vi "Data Storage - Pack Elements (B256).vi"(0 "data in":bool[](array[boolean]), 2 "reset":bool, 5 "input valid":bool, 7 "bit count":u16, 12 "ready for output (T)":bool=TRUE) -> (4 "data out":bool[](array[boolean]), 6 "output valid":bool, 14 "ready for input":bool)   [LabVIEW 2018, in "Streaming FPGA.lvlib"]
doc: "Packs arrays of booleans into arrays of 256 booleans.\n\nEach input array can have a different number of valid elements between 0 and 256, while the output array has always 256 valid elements. This VI reads <B>bit count</B> number of elements from the <B>data in</B> input array starting from the first element of the array, and returns them in arrays of 256 elements."
uses:
  Streaming FPGA.lvlib
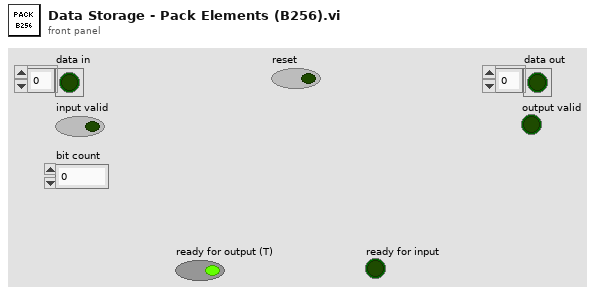
[diagram p1: front panel]
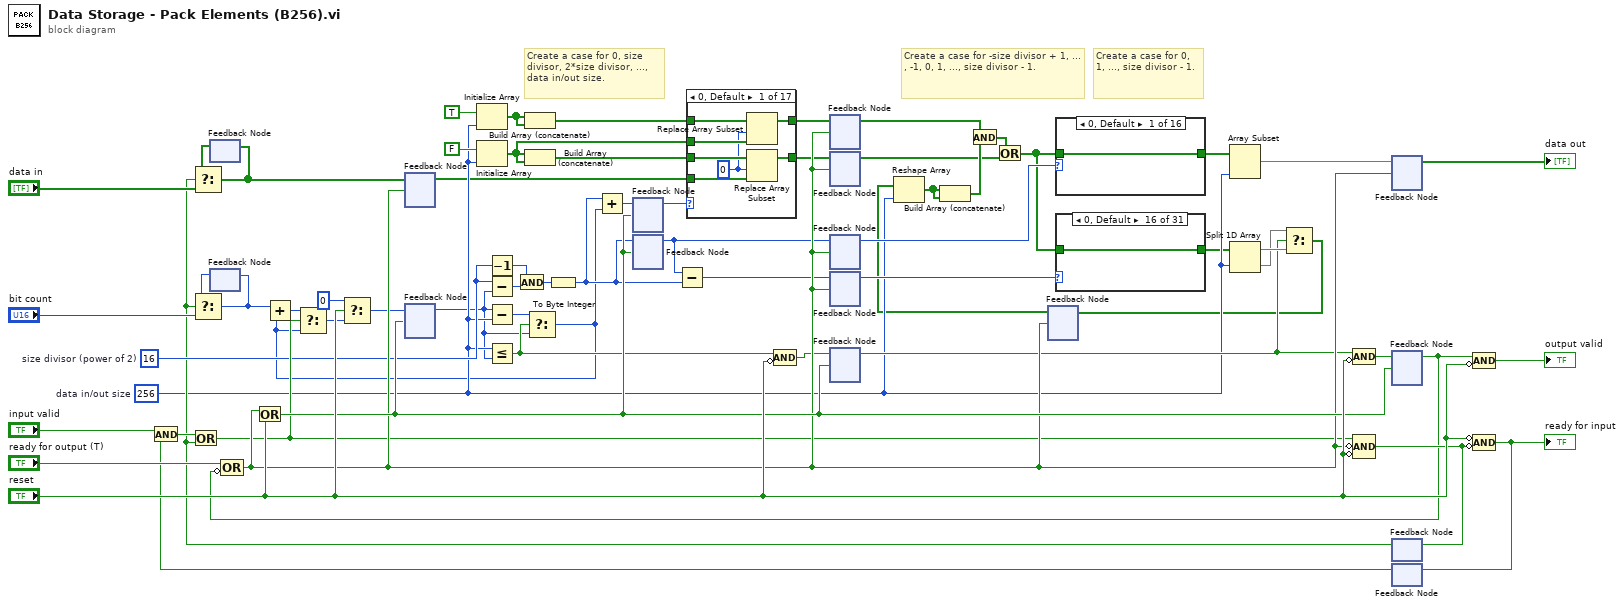
[diagram p0: block diagram]
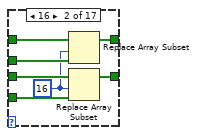
[diagram p2: hidden frame]
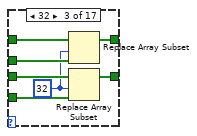
[diagram p3: hidden frame]
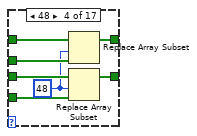
[diagram p4: hidden frame]
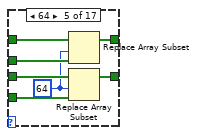
[diagram p5: hidden frame]
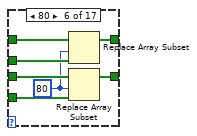
[diagram p6: hidden frame]
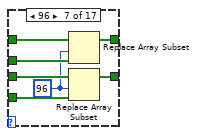
[diagram p7: hidden frame]
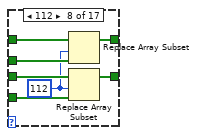
[diagram p8: hidden frame]
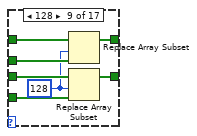
[diagram p9: hidden frame]
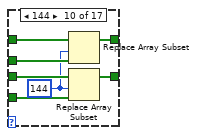
[diagram p10: hidden frame]
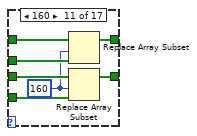
[diagram p11: hidden frame]
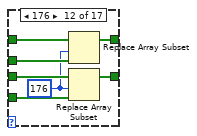
[diagram p12: hidden frame]
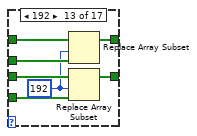
[diagram p13: hidden frame]
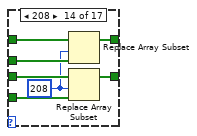
[diagram p14: hidden frame]
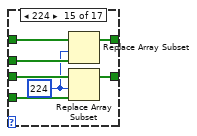
[diagram p15: hidden frame]
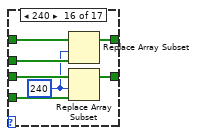
[diagram p16: hidden frame]
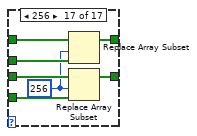
[diagram p17: hidden frame]
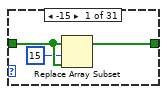
[diagram p18: hidden frame]
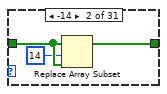
[diagram p19: hidden frame]
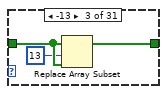
[diagram p20: hidden frame]
diagram:
  w52 = u16 16  # size divisor (power of 2)
  w27 = u16 256  # data in/out size
  # "Create a case for 0, 1, ..., size divisor - 1."
  # "Create a case for -size divisor + 1, ..., -1, 0, 1, ..., size divisor - 1."
  # "Create a case for 0, size divisor, 2*size divisor, ..., data in/out size."
  n1 = feedback #1() -> (w59:bool[])  [unwired: 1 in]
  n2 = feedback #2() -> (w56:u16)  [unwired: 1 in]
  n3 = feedback #3() -> (w4:bool[])  [unwired: 1 in]
  n4 = feedback #4() -> (w7:u16)  [unwired: 1 in]
  n5 = Initialize Array(TRUE ("element"), w27) -> (w24:bool[])
  n6 = Initialize Array(FALSE, w27) -> (w21:bool[])
  n7 = Decrement(x=w52) -> (x-1=w54:u16)
  n8 = Subtract(x=w52, y=w7) -> (x-y=w55:u16)
  n9 = Subtract(x=w7, y=w27) -> (x-y=w61:u16)
  n10 = Less Or Equal?(x=w27, y=w7) -> (x <= y?=w40:bool)
  n11 = And(x=w54, y=w55) -> (x .and. y?=w47:u16)
  n12 = Build Array (concatenate)(w24, w24) -> (w22:bool[])
  n13 = Build Array (concatenate)(w21, w21) -> (w23:bool[])
  n14 = Select(t=w61, s=w40, f=w7) -> (s? t:f=w6:u16)
  n15 = To Byte Integer(number=w47) -> (8bit integer=w12:i8)
  n16 = Add(x=w12, y=w6) -> (x+y=w11:u16)
  n17 = feedback #5() -> (w25:u16)  [unwired: 1 in]
  n18 = feedback #6() -> (w42:i8)  [unwired: 1 in]
  n19 = Subtract(x=w42, y=w12) -> (x-y=w44:i8)
  n20 = case shown="0, Default" w25 {
    tunnel: w23 -> [w72 w79 w86 w93 w100 w107 w114 w121 w128 w135 w142 w149 w156 w163 w170 w177 w184]
    tunnel: w4 -> [w71 w78 w85 w92 w99 w106 w113 w120 w127 w134 w141 w148 w155 w162 w169 w176 w183]
    tunnel: [w70 w77 w84 w91 w98 w105 w112 w119 w126 w133 w140 w147 w154 w161 w168 w175 w182] -> w20
    tunnel: w22 -> [w69 w76 w83 w90 w97 w104 w111 w118 w125 w132 w139 w146 w153 w160 w167 w174 w181]
    tunnel: w21 -> [w68 w75 w82 w89 w96 w103 w110 w117 w124 w131 w138 w145 w152 w159 w166 w173 w180]
    tunnel: [w66 w73 w80 w87 w94 w101 w108 w115 w122 w129 w136 w143 w150 w157 w164 w171 w178] -> w19
    frame 0, Default {
      w67 = 0 ("index")
      n21 = Replace Array Subset(array=w69, new element=w68, index=w67) -> (w66:bool[])
      n22 = Replace Array Subset(array=w72, new element=w71, index=w67) -> (w70:bool[])
    }
    frame 16 {
      w74 = 16 ("index")
      n23 = Replace Array Subset(array=w76, new element=w75, index=w74) -> (w73:bool[])
      n24 = Replace Array Subset(array=w79, new element=w78, index=w74) -> (w77:bool[])
    }
    frame 32 {
      w81 = 32 ("index")
      n25 = Replace Array Subset(array=w83, new element=w82, index=w81) -> (w80:bool[])
      n26 = Replace Array Subset(array=w86, new element=w85, index=w81) -> (w84:bool[])
    }
    frame 48 {
      w88 = 48 ("index")
      n27 = Replace Array Subset(array=w90, new element=w89, index=w88) -> (w87:bool[])
      n28 = Replace Array Subset(array=w93, new element=w92, index=w88) -> (w91:bool[])
    }
    frame 64 {
      w95 = 64 ("index")
      n29 = Replace Array Subset(array=w97, new element=w96, index=w95) -> (w94:bool[])
      n30 = Replace Array Subset(array=w100, new element=w99, index=w95) -> (w98:bool[])
    }
    frame 80 {
      w102 = 80 ("index")
      n31 = Replace Array Subset(array=w104, new element=w103, index=w102) -> (w101:bool[])
      n32 = Replace Array Subset(array=w107, new element=w106, index=w102) -> (w105:bool[])
    }
    frame 96 {
      w109 = 96 ("index")
      n33 = Replace Array Subset(array=w111, new element=w110, index=w109) -> (w108:bool[])
      n34 = Replace Array Subset(array=w114, new element=w113, index=w109) -> (w112:bool[])
    }
    frame 112 {
      w116 = 112 ("index")
      n35 = Replace Array Subset(array=w118, new element=w117, index=w116) -> (w115:bool[])
      n36 = Replace Array Subset(array=w121, new element=w120, index=w116) -> (w119:bool[])
    }
    frame 128 {
      w123 = 128 ("index")
      n37 = Replace Array Subset(array=w125, new element=w124, index=w123) -> (w122:bool[])
      n38 = Replace Array Subset(array=w128, new element=w127, index=w123) -> (w126:bool[])
    }
    frame 144 {
      w130 = 144 ("index")
      n39 = Replace Array Subset(array=w132, new element=w131, index=w130) -> (w129:bool[])
      n40 = Replace Array Subset(array=w135, new element=w134, index=w130) -> (w133:bool[])
    }
    frame 160 {
      w137 = 160 ("index")
      n41 = Replace Array Subset(array=w139, new element=w138, index=w137) -> (w136:bool[])
      n42 = Replace Array Subset(array=w142, new element=w141, index=w137) -> (w140:bool[])
    }
    frame 176 {
      w144 = 176 ("index")
      n43 = Replace Array Subset(array=w146, new element=w145, index=w144) -> (w143:bool[])
      n44 = Replace Array Subset(array=w149, new element=w148, index=w144) -> (w147:bool[])
    }
    frame 192 {
      w151 = 192 ("index")
      n45 = Replace Array Subset(array=w153, new element=w152, index=w151) -> (w150:bool[])
      n46 = Replace Array Subset(array=w156, new element=w155, index=w151) -> (w154:bool[])
    }
    frame 208 {
      w158 = 208 ("index")
      n47 = Replace Array Subset(array=w160, new element=w159, index=w158) -> (w157:bool[])
      n48 = Replace Array Subset(array=w163, new element=w162, index=w158) -> (w161:bool[])
    }
    frame 224 {
      w165 = 224 ("index")
      n49 = Replace Array Subset(array=w167, new element=w166, index=w165) -> (w164:bool[])
      n50 = Replace Array Subset(array=w170, new element=w169, index=w165) -> (w168:bool[])
    }
    frame 240 {
      w172 = 240 ("index")
      n51 = Replace Array Subset(array=w174, new element=w173, index=w172) -> (w171:bool[])
      n52 = Replace Array Subset(array=w177, new element=w176, index=w172) -> (w175:bool[])
    }
    frame 256 {
      w179 = 256 ("index")
      n53 = Replace Array Subset(array=w181, new element=w180, index=w179) -> (w178:bool[])
      n54 = Replace Array Subset(array=w184, new element=w183, index=w179) -> (w182:bool[])
    }
  }
  n55 = Compound Arithmetic op=AND(w40, invert "reset") -> (w13:bool)
  n56 = feedback #7() -> (w18:bool[])  [unwired: 1 in]
  n57 = feedback #8() -> (w16:bool[])  [unwired: 1 in]
  n58 = feedback #9() -> (w41:i8)  [unwired: 1 in]
  n59 = feedback #10() -> (w43:i8)  [unwired: 1 in]
  n60 = feedback #11() -> (w35:bool)  [unwired: 1 in]
  n61 = feedback #12() -> (w3:bool[])  [unwired: 1 in]
  n62 = Reshape Array(w3, w27) -> (w50:bool[])
  n63 = Build Array (concatenate)(w50, w50) -> (w17:bool[])
  n64 = And(x=w18, y=w17) -> (x .and. y?=w15:bool[])
  n65 = Or(x=w15, y=w16) -> (x .or. y?=w14:bool[])
  n66 = case shown="0, Default" w41 {
    tunnel: w14 -> [w185 w190 w195 w200 w205 w210 w215 w220 w225 w230 w235 w240 w245 w250 w255 w260]
    tunnel: [w185 w186 w191 w196 w201 w206 w211 w216 w221 w226 w231 w236 w241 w246 w251 w256] -> w49
    frame 0, Default {
    }
    frame 1 {
      n67 = Split 1D Array(array=w190, index=1) -> (first subarray=w187:bool[], second subarray=w188:bool[])
      n68 = Build Array (concatenate)(w188, w187) -> (w186:bool[])
    }
    frame 2 {
      n69 = Split 1D Array(array=w195, index=2) -> (first subarray=w192:bool[], second subarray=w193:bool[])
      n70 = Build Array (concatenate)(w193, w192) -> (w191:bool[])
    }
    frame 3 {
      n71 = Split 1D Array(array=w200, index=3) -> (first subarray=w197:bool[], second subarray=w198:bool[])
      n72 = Build Array (concatenate)(w198, w197) -> (w196:bool[])
    }
    frame 4 {
      n73 = Split 1D Array(array=w205, index=4) -> (first subarray=w202:bool[], second subarray=w203:bool[])
      n74 = Build Array (concatenate)(w203, w202) -> (w201:bool[])
    }
    frame 5 {
      n75 = Split 1D Array(array=w210, index=5) -> (first subarray=w207:bool[], second subarray=w208:bool[])
      n76 = Build Array (concatenate)(w208, w207) -> (w206:bool[])
    }
    frame 6 {
      n77 = Split 1D Array(array=w215, index=6) -> (first subarray=w212:bool[], second subarray=w213:bool[])
      n78 = Build Array (concatenate)(w213, w212) -> (w211:bool[])
    }
    frame 7 {
      n79 = Split 1D Array(array=w220, index=7) -> (first subarray=w217:bool[], second subarray=w218:bool[])
      n80 = Build Array (concatenate)(w218, w217) -> (w216:bool[])
    }
    frame 8 {
      n81 = Split 1D Array(array=w225, index=8) -> (first subarray=w222:bool[], second subarray=w223:bool[])
      n82 = Build Array (concatenate)(w223, w222) -> (w221:bool[])
    }
    frame 9 {
      n83 = Split 1D Array(array=w230, index=9) -> (first subarray=w227:bool[], second subarray=w228:bool[])
      n84 = Build Array (concatenate)(w228, w227) -> (w226:bool[])
    }
    frame 10 {
      n85 = Split 1D Array(array=w235, index=10) -> (first subarray=w232:bool[], second subarray=w233:bool[])
      n86 = Build Array (concatenate)(w233, w232) -> (w231:bool[])
    }
    frame 11 {
      n87 = Split 1D Array(array=w240, index=11) -> (first subarray=w237:bool[], second subarray=w238:bool[])
      n88 = Build Array (concatenate)(w238, w237) -> (w236:bool[])
    }
    frame 12 {
      n89 = Split 1D Array(array=w245, index=12) -> (first subarray=w242:bool[], second subarray=w243:bool[])
      n90 = Build Array (concatenate)(w243, w242) -> (w241:bool[])
    }
    frame 13 {
      n91 = Split 1D Array(array=w250, index=13) -> (first subarray=w247:bool[], second subarray=w248:bool[])
      n92 = Build Array (concatenate)(w248, w247) -> (w246:bool[])
    }
    frame 14 {
      n93 = Split 1D Array(array=w255, index=14) -> (first subarray=w252:bool[], second subarray=w253:bool[])
      n94 = Build Array (concatenate)(w253, w252) -> (w251:bool[])
    }
    frame 15 {
      n95 = Split 1D Array(array=w260, index=15) -> (first subarray=w257:bool[], second subarray=w258:bool[])
      n96 = Build Array (concatenate)(w258, w257) -> (w256:bool[])
    }
  }
  n97 = case shown="0, Default" w43 {
    tunnel: w14 -> [w262 w265 w268 w271 w274 w277 w280 w283 w286 w289 w292 w295 w298 w301 w304 w306 w311 w316 w321 w326 w331 w336 w341 w346 w351 w356 w361 w366 w371 w376 w381]
    tunnel: [w263 w266 w269 w272 w275 w278 w281 w284 w287 w290 w293 w296 w299 w302 w305 w306 w307 w312 w317 w322 w327 w332 w337 w342 w347 w352 w357 w362 w367 w372 w377] -> w1
    frame -15 {
      n98 = Replace Array Subset(array=w262, new element=w262, index=15) -> (w263:bool[])
    }
    frame -14 {
      n99 = Replace Array Subset(array=w265, new element=w265, index=14) -> (w266:bool[])
    }
    frame -13 {
      n100 = Replace Array Subset(array=w268, new element=w268, index=13) -> (w269:bool[])
    }
    frame -12 {
      n101 = Replace Array Subset(array=w271, new element=w271, index=12) -> (w272:bool[])
    }
    frame -11 {
      n102 = Replace Array Subset(array=w274, new element=w274, index=11) -> (w275:bool[])
    }
    frame -10 {
      n103 = Replace Array Subset(array=w277, new element=w277, index=10) -> (w278:bool[])
    }
    frame -9 {
      n104 = Replace Array Subset(array=w280, new element=w280, index=9) -> (w281:bool[])
    }
    frame -8 {
      n105 = Replace Array Subset(array=w283, new element=w283, index=8) -> (w284:bool[])
    }
    frame -7 {
      n106 = Replace Array Subset(array=w286, new element=w286, index=7) -> (w287:bool[])
    }
    frame -6 {
      n107 = Replace Array Subset(array=w289, new element=w289, index=6) -> (w290:bool[])
    }
    frame -5 {
      n108 = Replace Array Subset(array=w292, new element=w292, index=5) -> (w293:bool[])
    }
    frame -4 {
      n109 = Replace Array Subset(array=w295, new element=w295, index=4) -> (w296:bool[])
    }
    frame -3 {
      n110 = Replace Array Subset(array=w298, new element=w298, index=3) -> (w299:bool[])
    }
    frame -2 {
      n111 = Replace Array Subset(array=w301, new element=w301, index=2) -> (w302:bool[])
    }
    frame -1 {
      n112 = Replace Array Subset(array=w304, new element=w304, index=1) -> (w305:bool[])
    }
    frame 0, Default {
    }
    frame 1 {
      n113 = Split 1D Array(array=w311, index=1) -> (first subarray=w308:bool[], second subarray=w309:bool[])
      n114 = Build Array (concatenate)(w309, w308) -> (w307:bool[])
    }
    frame 2 {
      n115 = Split 1D Array(array=w316, index=2) -> (first subarray=w313:bool[], second subarray=w314:bool[])
      n116 = Build Array (concatenate)(w314, w313) -> (w312:bool[])
    }
    frame 3 {
      n117 = Split 1D Array(array=w321, index=3) -> (first subarray=w318:bool[], second subarray=w319:bool[])
      n118 = Build Array (concatenate)(w319, w318) -> (w317:bool[])
    }
    frame 4 {
      n119 = Split 1D Array(array=w326, index=4) -> (first subarray=w323:bool[], second subarray=w324:bool[])
      n120 = Build Array (concatenate)(w324, w323) -> (w322:bool[])
    }
    frame 5 {
      n121 = Split 1D Array(array=w331, index=5) -> (first subarray=w328:bool[], second subarray=w329:bool[])
      n122 = Build Array (concatenate)(w329, w328) -> (w327:bool[])
    }
    frame 6 {
      n123 = Split 1D Array(array=w336, index=6) -> (first subarray=w333:bool[], second subarray=w334:bool[])
      n124 = Build Array (concatenate)(w334, w333) -> (w332:bool[])
    }
    frame 7 {
      n125 = Split 1D Array(array=w341, index=7) -> (first subarray=w338:bool[], second subarray=w339:bool[])
      n126 = Build Array (concatenate)(w339, w338) -> (w337:bool[])
    }
    frame 8 {
      n127 = Split 1D Array(array=w346, index=8) -> (first subarray=w343:bool[], second subarray=w344:bool[])
      n128 = Build Array (concatenate)(w344, w343) -> (w342:bool[])
    }
    frame 9 {
      n129 = Split 1D Array(array=w351, index=9) -> (first subarray=w348:bool[], second subarray=w349:bool[])
      n130 = Build Array (concatenate)(w349, w348) -> (w347:bool[])
    }
    frame 10 {
      n131 = Split 1D Array(array=w356, index=10) -> (first subarray=w353:bool[], second subarray=w354:bool[])
      n132 = Build Array (concatenate)(w354, w353) -> (w352:bool[])
    }
    frame 11 {
      n133 = Split 1D Array(array=w361, index=11) -> (first subarray=w358:bool[], second subarray=w359:bool[])
      n134 = Build Array (concatenate)(w359, w358) -> (w357:bool[])
    }
    frame 12 {
      n135 = Split 1D Array(array=w366, index=12) -> (first subarray=w363:bool[], second subarray=w364:bool[])
      n136 = Build Array (concatenate)(w364, w363) -> (w362:bool[])
    }
    frame 13 {
      n137 = Split 1D Array(array=w371, index=13) -> (first subarray=w368:bool[], second subarray=w369:bool[])
      n138 = Build Array (concatenate)(w369, w368) -> (w367:bool[])
    }
    frame 14 {
      n139 = Split 1D Array(array=w376, index=14) -> (first subarray=w373:bool[], second subarray=w374:bool[])
      n140 = Build Array (concatenate)(w374, w373) -> (w372:bool[])
    }
    frame 15 {
      n141 = Split 1D Array(array=w381, index=15) -> (first subarray=w378:bool[], second subarray=w379:bool[])
      n142 = Build Array (concatenate)(w379, w378) -> (w377:bool[])
    }
  }
  n143 = Array Subset(array=w49, length=w27) -> (w48:bool[])  [unwired: 1 in]
  n144 = Split 1D Array(array=w1, index=w27) -> (first subarray=w46:bool[], second subarray=w45:bool[])
  n145 = Select(t=w45, s=w35, f=w46) -> (s? t:f=w2:bool[])
  n146 = Compound Arithmetic op=AND(w35, invert "reset") -> (w38:bool)
  n147 = feedback #13() -> (→"data out":bool[])  [unwired: 1 in]
  n148 = feedback #14() -> (w29:bool)  [unwired: 1 in]
  n149 = Compound Arithmetic op=OR("ready for output (T)", invert w29) -> (w63:bool)
  n150 = Or(x=w63, y="reset") -> (x .or. y?=w64:bool)
  n151 = feedback-in #5(w11, w64) -> ()
  n152 = feedback-in #6(w12, w64) -> ()
  n153 = feedback-in #7(w19, w63) -> ()
  n154 = feedback-in #8(w20, w63) -> ()
  n155 = feedback-in #9(w42, w63) -> ()
  n156 = feedback-in #10(w44, w63) -> ()
  n157 = feedback-in #11(w13, w64) -> ()
  n158 = feedback-in #12(w2, w63) -> ()
  n159 = feedback-in #13(w48, w63) -> ()
  n160 = feedback-in #14(w38, w64) -> ()
  n161 = feedback #15() -> (w30:bool)  [unwired: 1 in]
  n162 = Select(t=w59, s=w30, f="data in") -> (s? t:f=w5:bool[])
  n163 = Select(t=w56, s=w30, f="bit count") -> (s? t:f=w57:u16)
  n164 = feedback-in #1(w5) -> ()
  n165 = feedback-in #2(w57) -> ()
  n166 = Add(x=w57, y=w6) -> (x+y=w51:u16)
  n167 = feedback-in #3(w5, w63) -> ()
  n168 = feedback #16() -> (w32:bool)  [unwired: 1 in]
  n169 = And(x="input valid", y=w32) -> (x .and. y?=w39:bool)
  n170 = Or(x=w39, y=w30) -> (x .or. y?=w62:bool)
  n171 = Select(t=w51, s=w62, f=w6) -> (s? t:f=w10:u16)
  n172 = Select(t=u16 0, s="reset", f=w10) -> (s? t:f=w8:u16)
  n173 = feedback-in #4(w8, w64) -> ()
  n174 = Compound Arithmetic op=AND(w62, invert w63, invert "reset") -> (w31:bool)
  n175 = feedback-in #15(w31) -> ()
  n176 = Compound Arithmetic op=AND(w29, invert "reset") -> (→"output valid":bool)
  n177 = Compound Arithmetic op=AND(invert "reset", invert w31) -> (w33:bool)
  "ready for input" <- w33
  n178 = feedback-in #16(w33) -> ()
